vi "ShooterBallVelocityCompensation2.vi"(9 "Shooter Upper Speed Goal":dbl, 10 "Shooter Lower Speed Goal":dbl) -> (2 "Compensated Speed Goal":dbl)   [LabVIEW 2020]
uses:
  robotconstants.vi
  sensordata.vi
panel:
  in  "Ball Slip Tuning Parameter":dbl=2.0
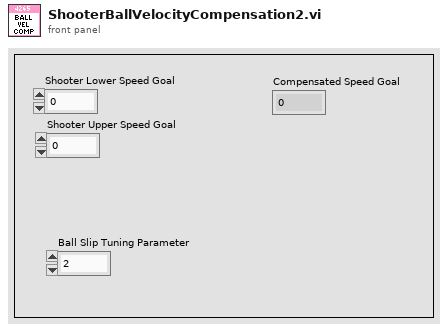
[diagram p1: front panel]
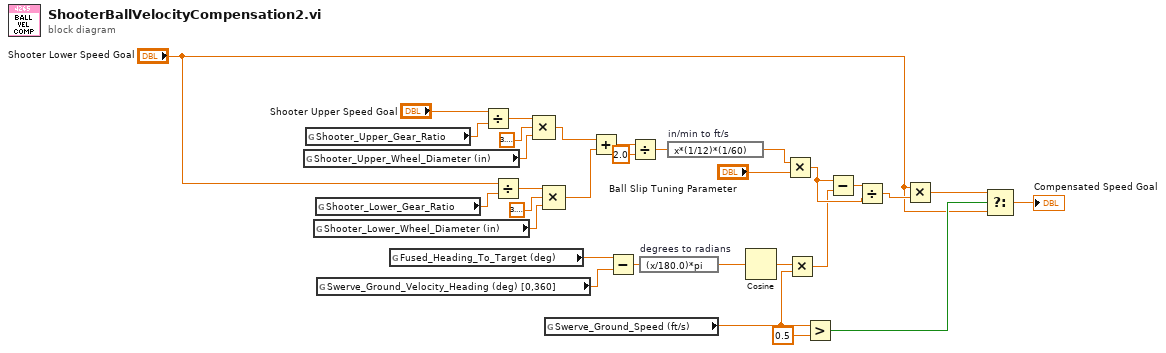
[diagram p0: block diagram]
diagram:
  n1 = global read "robotconstants.vi" "Shooter_Upper_Wheel_Diameter (in)"() -> (w27:dbl)
  n2 = global read "robotconstants.vi" "Shooter_Upper_Gear_Ratio"() -> (w30:dbl)
  n3 = global read "robotconstants.vi" "Shooter_Lower_Wheel_Diameter (in)"() -> (w22:dbl)
  n4 = global read "robotconstants.vi" "Shooter_Lower_Gear_Ratio"() -> (w25:dbl)
  n5 = global read "sensordata.vi" "Swerve_Ground_Velocity_Heading (deg) [0,360]"() -> (w13:dbl)
  n6 = global read "sensordata.vi" "Fused_Heading_To_Target (deg)"() -> (w31:dbl)
  n7 = Divide(x="Shooter Upper Speed Goal", y=w30) -> (x/y=w29:dbl)
  n8 = Divide(x="Shooter Lower Speed Goal", y=w25) -> (x/y=w24:dbl)
  n9 = Compound Arithmetic op=MULTIPLY(w29, 3.141592653589793, w27) -> (w26:dbl)
  n10 = Compound Arithmetic op=MULTIPLY(w24, 3.141592653589793, w22) -> (w21:dbl)
  n11 = global read "sensordata.vi" "Swerve_Ground_Speed (ft/s)"() -> (w7:dbl)
  n12 = Add(x=w26, y=w21) -> (x+y=w20:dbl)
  n13 = Subtract(x=w31, y=w13) -> (x-y=w12:dbl)
  n14 = Divide(x=w20, y=2.0) -> (x/y=w18:dbl)
  n15 = expression code="(x/180.0)*pi" "degrees to radians"(w12) -> (w11:dbl)
  n16 = expression code="x*(1/12)*(1/60)" "in/min to ft/s"(w18) -> (w17:dbl)
  n17 = Cosine(x=w11) -> (cos(x)=w10:dbl)
  n18 = Multiply(x=w17, y="Ball Slip Tuning Parameter") -> (x*y=w14:dbl)
  n19 = Multiply(x=w10, y=w7) -> (x*y=w9:dbl)
  n20 = Greater?(x=w7, y=0.5) -> (0:w5:bool)
  n21 = Subtract(x=w14, y=w9) -> (x-y=w15:dbl)
  n22 = Divide(x=w15, y=w14) -> (x/y=w8:dbl)
  n23 = Multiply(x="Shooter Lower Speed Goal", y=w8) -> (x*y=w4:dbl)
  n24 = Select(t=w4, s=w5, f="Shooter Lower Speed Goal") -> (s? t:f=→"Compensated Speed Goal":dbl)
